vi "viewerDisplay.vi"(8 "error in (no error)":errorcluster, 11 "ImageStreamViewer in":refnum<class "ImageStreamViewer.lvclass">) -> (0 "error out":errorcluster, 3 "ImageStreamViewer out":refnum<class "ImageStreamViewer.lvclass">)   [LabVIEW 2009, in "Views.lvlib" / "Camera.lvlib" / "ImageStreamViewer.lvclass"]
uses:
  ImageStreamViewer.lvclass
  ImageStreamViewer.lvclass/ImageStreamViewer.ctl
panel:
  in  "stop":bool
  out "y profile":cluster{"Pixels Line":sgl[], i32[]}(graph)
  out "X Profile":cluster{"x0":sgl, "dx":sgl, "Pixels Line":sgl[]}(graph)
  in  "Scrollbar":i32(c297)
  out "Path":path
  out "Image":T1(plugin-control)
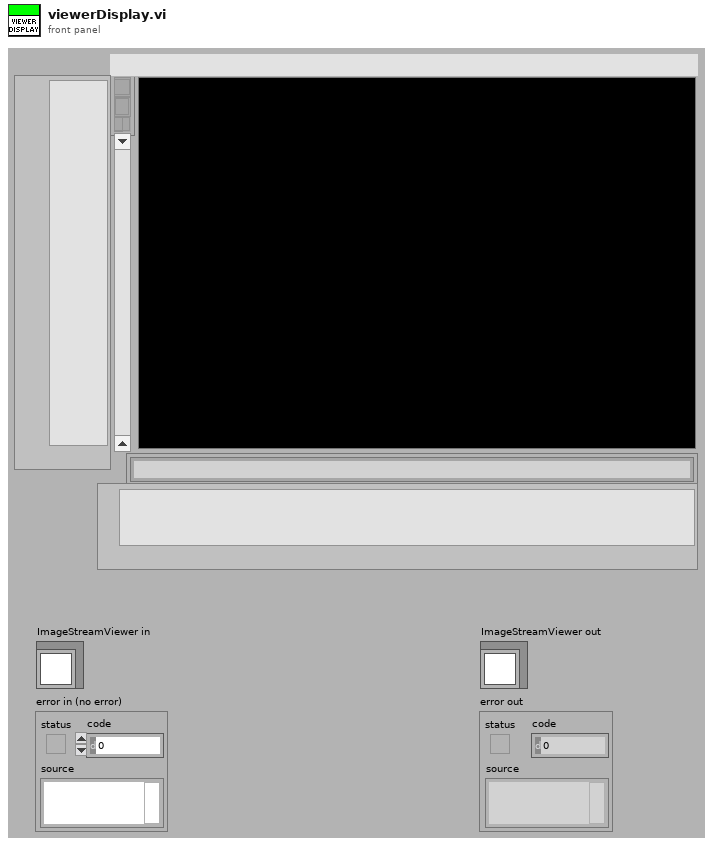
[diagram p1: front panel]
types:
  T1 = typedef "IMAQ Image.ctl" = refnum<image>
  T2 = typedef "LVPoint32TypeDef.ctl" = cluster{"Horizontal":i32, "Vertical":i32}
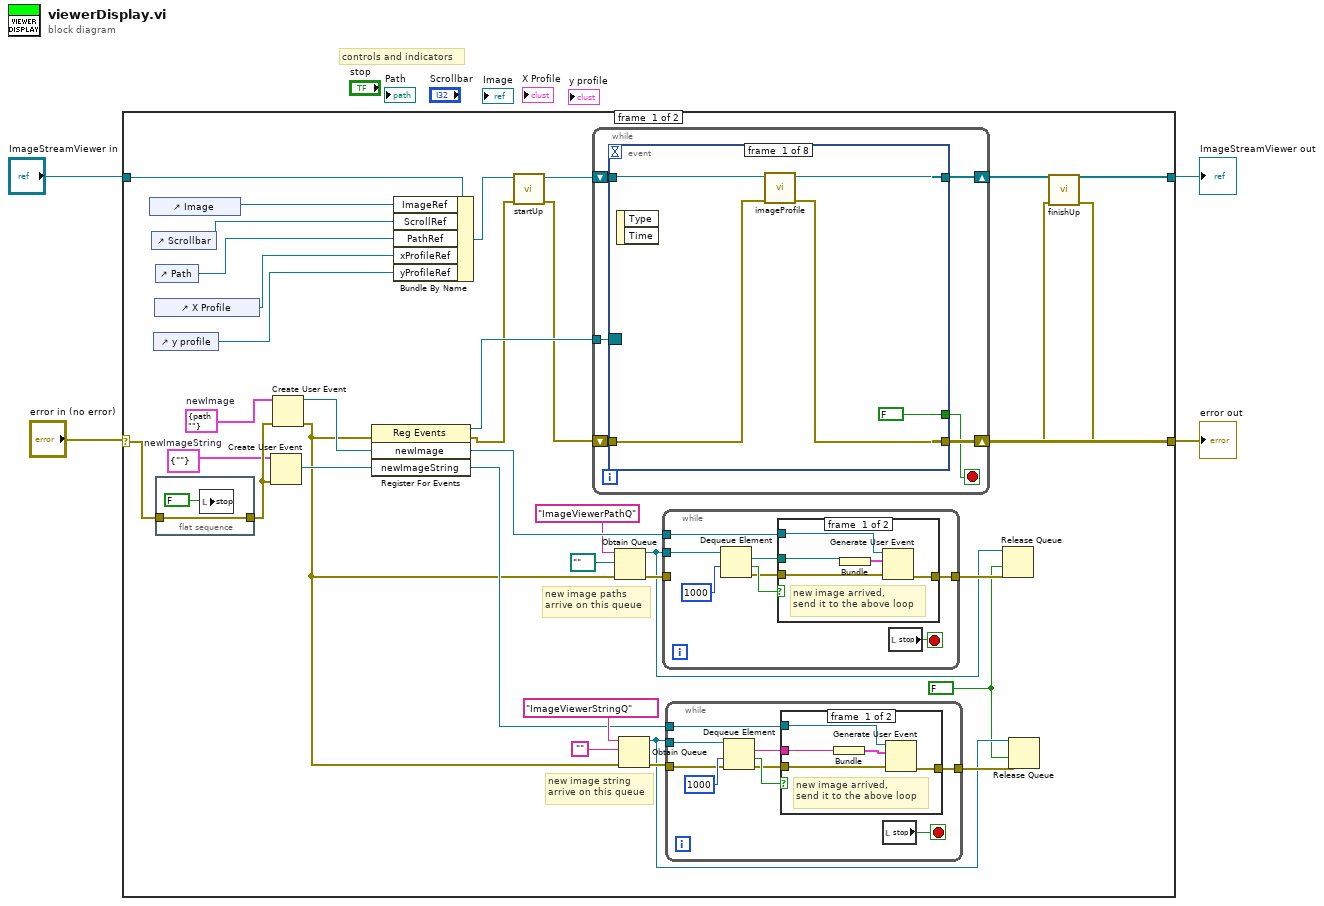
[diagram p0: block diagram]
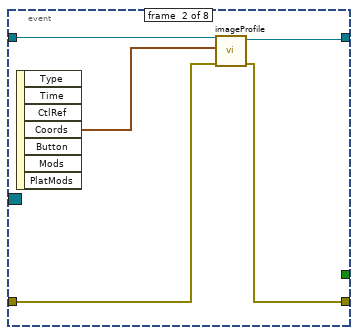
[diagram p4: hidden frame]
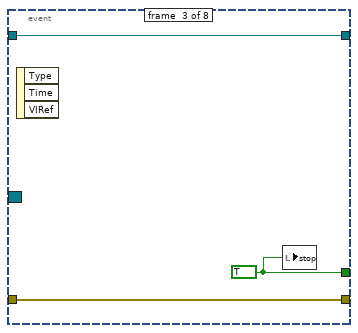
[diagram p5: hidden frame]
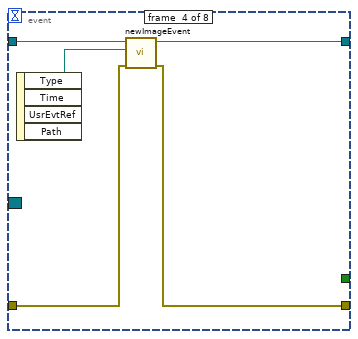
[diagram p6: hidden frame]
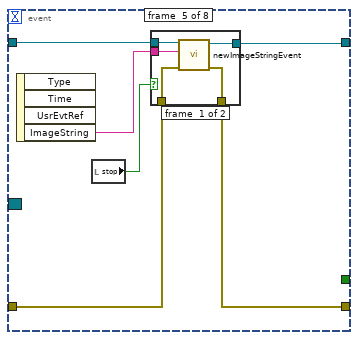
[diagram p7: hidden frame]
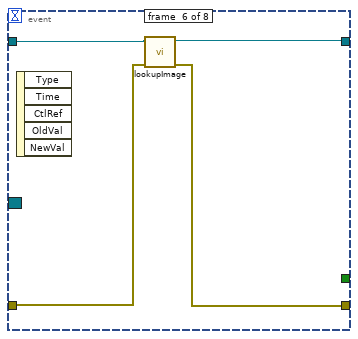
[diagram p9: hidden frame]
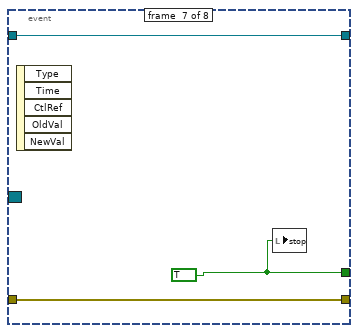
[diagram p10: hidden frame]
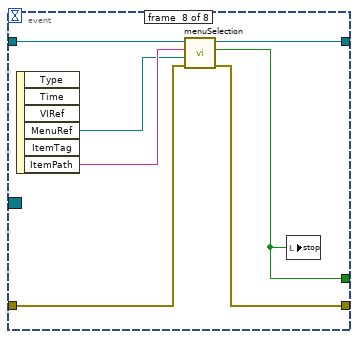
[diagram p11: hidden frame]
diagram:
  # "controls and indicators"
  n1 = case shown="No Error" "error in (no error)" {
    selector: "error in (no error)" -> [w31 w121]
    tunnel: [w15 w121] -> w3
    tunnel: [w17 w120] -> w1
    tunnel: "ImageStreamViewer in" -> [w30 w120]
    frame #0 {
      w10 = FALSE
      w20 = cluster{"ImageString":string} {"ImageString"=""}  # newImageString
      w36 = cluster{"Path":path} {"Path"=path ""}  # newImage
      # "new image string\narrive on this queue"
      # "new image paths\narrive on this queue"
      n2 = control-ref of="Image"() -> (w29:refnum<vi>)
      n3 = control-ref of="Scrollbar"() -> (w28:refnum<vi>)
      n4 = control-ref of="y profile"() -> (w25:refnum<vi>)
      n5 = control-ref of="X Profile"() -> (w26:refnum<vi>)
      n6 = control-ref of="Path"() -> (w27:refnum<vi>)
      n7 = flat-sequence {
        tunnel: w31 -> [w53]
        tunnel: [w53] -> w21
        frame #0 {
          n8 = local write "stop"(FALSE) -> ()
        }
      }
      n9 = Create User Event(user event datatype=w20, error in=w21) -> (user event=w19:refnum<user-event>)  [unwired: 1 out]
      n10 = Create User Event(user event datatype=w36, error in=w21) -> (user event=w35:refnum<user-event>, error out=w5:errorcluster)
      n11 = register-events(error in=w5, w35, w19) -> (reference out=w37:refnum<event-registration>, error out=w7:errorcluster)  [unwired: 1 in]
      n12 = Bundle By Name(cluster=w30, "ImageRef"=w29, "ScrollRef"=w28, "PathRef"=w27, "xProfileRef"=w26, "yProfileRef"=w25) -> (w9:refnum<class "ImageStreamViewer.lvclass">)
      n13 = call "startUp.vi"("error in (no error)"=w7, "ImageStreamViewer in"=w9) -> ("error out"=w6:errorcluster, "ImageStreamViewer out"=w8:refnum<class "ImageStreamViewer.lvclass">)  [unwired: 8 in]
      n14 = while {
        shift-right: [w72] -> w18
        shift-left: w8 -> [w74]
        shift-right: [w71] -> w16
        shift-left: w6 -> [w73]
        tunnel: w37 -> [w69]
        stop <- w70 stop-if-true
        n15 = event shown="[7] Menu Selection (User)" {
          selector: w69 -> [_ _ _ _ _ _ _ _]
          dyn-events: _ -> [_ _ _ _ _ _ _ _]
          timeout: _ -> [_ _ _ _ _ _ _ _]
          tunnel: w74 -> [w78 w84 w87 w92 w98 w109 w110 w119]
          tunnel: w73 -> [w76 w82 w85 w89 w95 w107 w112 w117]
          tunnel: [w77 w83 w87 w91 w97 w108 w110 w118] -> w72
          tunnel: [w75 w81 w85 w88 w94 w106 w112 w116] -> w71
          tunnel: [FALSE _ w86 _ _ _ w111 w114] -> w70
          event #0 {
            n16 = event-data() -> ()  [unwired: 1 in, 2 out]
            n17 = call "imageProfile.vi"("error in (no error)"=w76, "ImageStreamViewer in"=w78) -> ("error out"=w75:errorcluster, "ImageStreamViewer out"=w77:refnum<class "ImageStreamViewer.lvclass">)  [unwired: 8 in]
          }
          event #1 {
            n18 = event-data() -> ("Coords"=w80:T2)  [unwired: 1 in, 6 out]
            n19 = call "imageProfile.vi"("error in (no error)"=w82, "Point"=w80, "ImageStreamViewer in"=w84) -> ("error out"=w81:errorcluster, "ImageStreamViewer out"=w83:refnum<class "ImageStreamViewer.lvclass">)  [unwired: 7 in]
          }
          event #2 {
            w86 = TRUE
            n20 = event-data() -> ()  [unwired: 1 in, 3 out]
            n21 = local write "stop"(w86) -> ()
          }
          event #3 {
            n22 = event-data() -> ("Path"=w90:path)  [unwired: 1 in, 3 out]
            n23 = call "newImageEvent.vi"("error in (no error)"=w89, "Path"=w90, "ImageStreamViewer in"=w92) -> ("error out"=w88:errorcluster, "ImageStreamViewer out"=w91:refnum<class "ImageStreamViewer.lvclass">)  [unwired: 7 in]
          }
          event #4 {
            n24 = event-data() -> ("ImageString"=w96:string)  [unwired: 1 in, 3 out]
            n25 = local read "stop"() -> (w93:bool)
            n26 = case shown="False" w93 {
              tunnel: w98 -> [w103 w105]
              tunnel: [w102 w105] -> w97
              tunnel: w96 -> [w101 _]
              tunnel: w95 -> [w100 w104]
              tunnel: [w99 w104] -> w94
              frame #0 {
                n27 = call "newImageStringEvent.vi"("error in (no error)"=w100, "ImageString"=w101, "ImageStreamViewer in"=w103) -> ("error out"=w99:errorcluster, "ImageStreamViewer out"=w102:refnum<class "ImageStreamViewer.lvclass">)  [unwired: 7 in]
              }
              frame #1 {
              }
            }
          }
          event #5 {
            n28 = event-data() -> ()  [unwired: 1 in, 5 out]
            n29 = call "lookupImage.vi"("error in (no error)"=w107, "ImageStreamViewer in"=w109) -> ("error out"=w106:errorcluster, "ImageStreamViewer out"=w108:refnum<class "ImageStreamViewer.lvclass">)  [unwired: 8 in]
          }
          event #6 {
            w111 = TRUE
            n30 = event-data() -> ()  [unwired: 1 in, 5 out]
            n31 = local write "stop"(w111) -> ()
          }
          event #7 {
            n32 = event-data() -> ("MenuRef"=w113:refnum<k9>, "ItemPath"=w115:string)  [unwired: 1 in, 4 out]
            n33 = call "menuSelection.vi"("error in (no error)"=w117, "MenuRef"=w113, "itemPath"=w115, "ImageStreamViewer in"=w119) -> ("error out"=w116:errorcluster, "close"=w114:bool, "ImageStreamViewer out"=w118:refnum<class "ImageStreamViewer.lvclass">)  [unwired: 5 in]
            n34 = local write "stop"(w114) -> ()
          }
        }
      }
      n35 = Obtain Queue(name (unnamed)="ImageViewerPathQ", element data type=path "", error in (no error)=w5) -> (queue out=w11:refnum<queue>, error out=w32:errorcluster)  [unwired: 2 in, 1 out]
      n36 = Obtain Queue(name (unnamed)="ImageViewerStringQ", element data type="", error in (no error)=w5) -> (queue out=w13:refnum<queue>, error out=w22:errorcluster)  [unwired: 2 in, 1 out]
      n37 = while {
        tunnel: w35 -> [w57]
        tunnel: w11 -> [w62]
        tunnel: w32 -> [_]
        tunnel: [w56] -> w12
        stop <- w55 stop-if-true
        n38 = Dequeue Element(queue=w62, timeout in ms (-1)=1000) -> (element=w59:path, timed out?=w60:bool, error out=w58:errorcluster)  [unwired: 1 in, 1 out]
        n39 = case shown="False" w60 {
          tunnel: w59 -> [w64 _]
          tunnel: w58 -> [w67 w68]
          tunnel: w57 -> [w66 _]
          tunnel: [w63 w68] -> w56
          frame #0 {
            # "new image arrived, \nsend it to the above loop"
            n40 = Bundle(w64) -> (w65:cluster{path})  [unwired: 1 in]
            n41 = Generate User Event(user event=w66, event data cluster=w65, error in=w67) -> (error out=w63:errorcluster)  [unwired: 1 out]
          }
          frame #1 {
            # "timeout"
          }
        }
        n42 = local read "stop"() -> (w55:bool)
      }
      n43 = while {
        tunnel: w19 -> [w43]
        tunnel: [w42] -> w14
        tunnel: w22 -> [w39]
        tunnel: w13 -> [w38]
        stop <- w41 stop-if-true
        n44 = Dequeue Element(queue=w38, timeout in ms (-1)=1000, error in (no error)=w39) -> (element=w40:string, timed out?=w45:bool, error out=w44:errorcluster)  [unwired: 1 out]
        n45 = case shown="False" w45 {
          tunnel: w44 -> [w51 w52]
          tunnel: w43 -> [w50 _]
          tunnel: [w49 w52] -> w42
          tunnel: w40 -> [w47 _]
          frame #0 {
            # "new image arrived, \nsend it to the above loop"
            n46 = Bundle(w47) -> (w48:cluster{string})  [unwired: 1 in]
            n47 = Generate User Event(user event=w50, event data cluster=w48, error in=w51) -> (error out=w49:errorcluster)  [unwired: 1 out]
          }
          frame #1 {
            # "timeout"
          }
        }
        n48 = local read "stop"() -> (w41:bool)
      }
      n49 = Release Queue(queue=w11, force destroy? (F)=w10, error in (no error)=w12) -> ()  [unwired: 3 out]
      n50 = Release Queue(queue=w13, force destroy? (F)=w10, error in (no error)=w14) -> ()  [unwired: 3 out]
      n51 = call "finishUp.vi"("error in (no error)"=w16, "ImageStreamViewer in"=w18) -> ("error out"=w15:errorcluster, "ImageStreamViewer out"=w17:refnum<class "ImageStreamViewer.lvclass">)  [unwired: 8 in]
    }
    frame #1 {
    }
  }
  "error out" <- w3
  "ImageStreamViewer out" <- w1
